vi "Write Component Root Path.vi"(8 "error in (no error)":errorcluster, 10 "Component Definition ini Path":path, 11 "Commit in":refnum<class "Commit.lvclass">) -> (0 "error out":errorcluster, 3 "Commit out":refnum<class "Commit.lvclass">)   [LabVIEW 2017, in "CL_G3_VIComponentBuilder.lvlib" / "Commit.lvclass"]
uses:
  Commit.lvclass
  Commit.lvclass/Commit.ctl
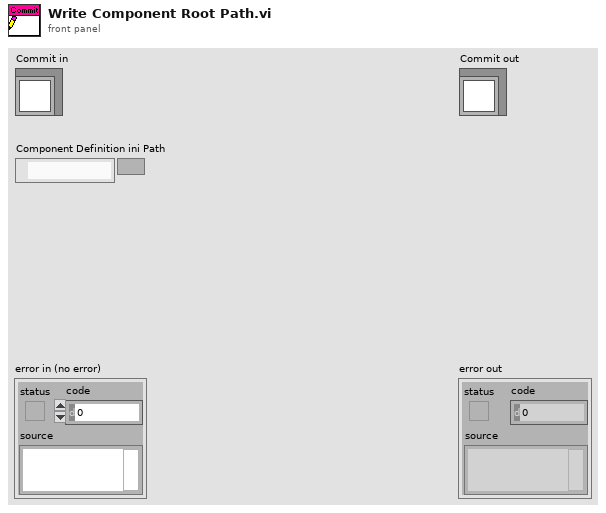
[diagram p1: front panel]
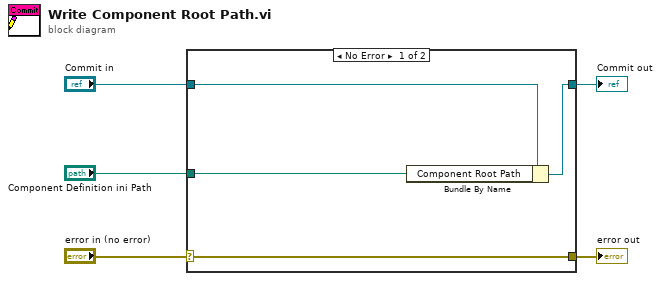
[diagram p0: block diagram]
diagram:
  n1 = case shown="No Error" "error in (no error)" {
    selector: "error in (no error)" -> [w9 w10]
    tunnel: [w9 w10] -> w4
    tunnel: [w7 w11] -> w2
    tunnel: "Commit in" -> [w8 w11]
    tunnel: "Component Definition ini Path" -> [w6 _]
    frame No Error {
      n2 = Bundle By Name(cluster=w8, "Component Root Path"=w6) -> (w7:refnum<class "Commit.lvclass">)
    }
    frame Error {
    }
  }
  "error out" <- w4
  "Commit out" <- w2
